vi "__anritsu_get_data_collection_time.vi"(2 "error in":errorcluster) -> (0 "error out":errorcluster, 1 "Measurment time (s)":dbl=0.493)   [LabVIEW 2013]
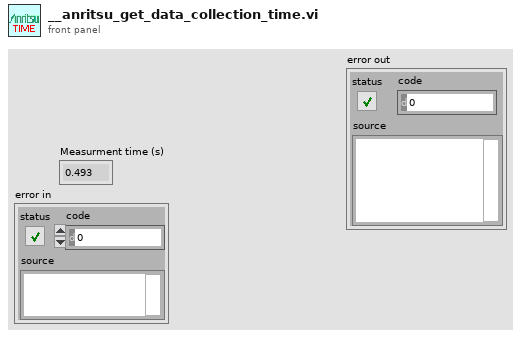
[diagram p1: front panel]
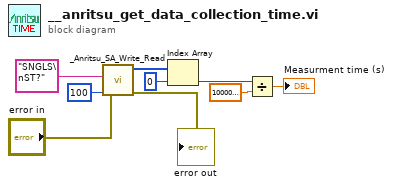
[diagram p0: block diagram]
diagram:
  n1 = call "_Anritsu_SA_Write_Read.vi"("bytes to read"=100, "error in (no error)"="error in", "Comand"="SNGLS\nST?") -> ("error out"=→"error out":errorcluster, "Data out"=w8:i32[])  [unwired: 3 in]
  n2 = Index Array(array=w8, index=0) -> (element=w5:i32)
  n3 = Divide(x=w5, y=1000000.0) -> (x/y=→"Measurment time (s)":dbl)
